vi "Shutdown.vi"(8 "error in (no error)":errorcluster, 11 "CLI in":refnum<class "CLI.lvclass">) -> (0 "error out":errorcluster, 3 "CLI out":refnum<class "CLI.lvclass">)   [LabVIEW 2020, in "neg-pkg-cli.lvlib" / "CLI.lvclass"]
uses:
  CLI.lvclass
  CLI.lvclass/CLI.ctl
  MGI Console/Source/Console/Console.lvclass
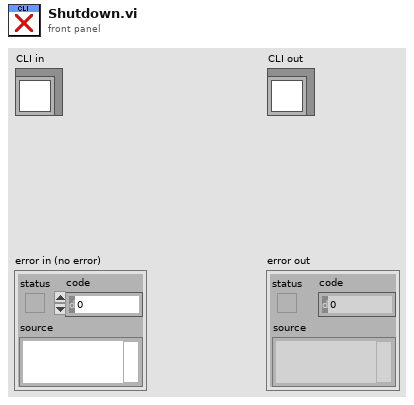
[diagram p1: front panel]
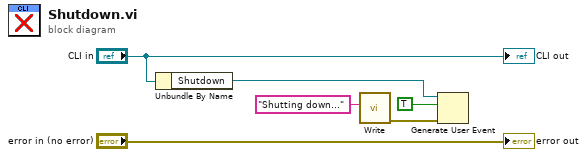
[diagram p0: block diagram]
diagram:
  n1 = Unbundle By Name("CLI in") -> ("Shutdown"=w4:refnum<user-event>)
  n2 = call "Write.vi"("String"="Shutting down...") -> ("error out"=w1:errorcluster)  [unwired: 10 in]
  n3 = Generate User Event(user event=w4, event data cluster=TRUE ("event data"), error in=w1) -> ()  [unwired: 1 in, 2 out]
  "error out" <- "error in (no error)"
  "CLI out" <- "CLI in"
